vi "TabShow.vi"(10 "index":i32, 11 "Buttons":T1) -> (3 "error out":errorcluster)   [LabVIEW 2019]
uses:
  TypeDef/#TypeDef_Buttons.ctl
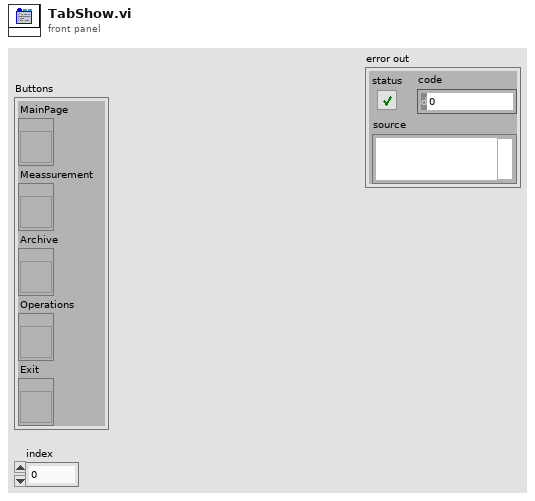
[diagram p1: front panel]
types:
  T1 = typedef "#TypeDef_Buttons.ctl" = cluster{"MainPage":refnum<vi>, "Meassurement":refnum<vi>, "Archive":refnum<vi>, "Operations":refnum<vi>, "Exit":refnum<vi>}
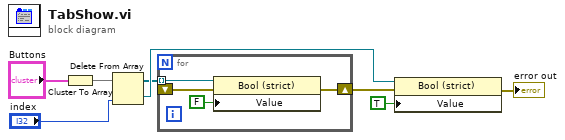
[diagram p0: block diagram]
diagram:
  n1 = Cluster To Array(cluster="Buttons") -> (array=w6:refnum<vi>[])
  n2 = Delete From Array(array=w6, index="index") -> (deleted portion=w8:refnum<vi>, array with subset deleted=w4:refnum<vi>[])  [unwired: 1 in]
  n3 = for {
    tunnel: w4 -> [w9] mode=indexing
    shift-right: [w11] -> w5
    shift-left: _ -> [w10]
    n4 = property class="Bool (strict)"(reference=w9, error in=w10, "Value"=FALSE) -> (error out=w11:errorcluster)  [unwired: 1 out]
  }
  n5 = property class="Bool (strict)"(reference=w8, error in=w5, "Value"=TRUE) -> (error out=→"error out":errorcluster)  [unwired: 1 out]
